vi "Read TDMS Double.vi"(8 "error in (no error)":errorcluster, 9 "channel name(s) in":string, 10 "offset (0)":i64, 11 "file path":path) -> (0 "error out":errorcluster, 3 "Data":dbl[](array[numeric]))   [LabVIEW 2014]
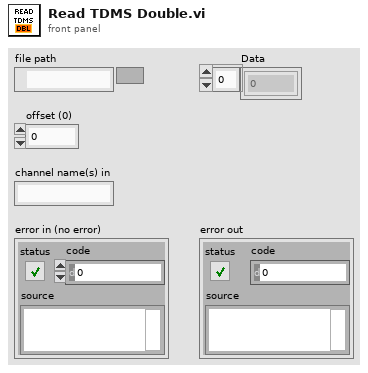
[diagram p1: front panel]
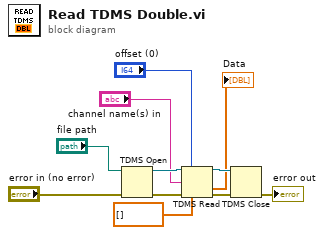
[diagram p0: block diagram]
diagram:
  n1 = TDMS Open(8:"error in (no error)", 11:"file path") -> (0:w11:errorcluster, 3:w10:refnum<k34>)  [unwired: 5 in]
  n2 = TDMS Read(0:w10, 1:"offset (0)", 7:"channel name(s) in", 11:w11, 12:dbl[] []) -> (4:w6:refnum<k34>, 10:→"Data":dbl[], 15:w5:errorcluster)  [unwired: 3 in, 3 out]
  n3 = TDMS Close(8:w5, 11:w6) -> (0:→"error out":errorcluster)  [unwired: 1 out]
